vi "Init.vi"(8 "error in (no error)":errorcluster, 10 "RIO Device":T1="RIO0", 11 "AODAcq in":refnum<class "AODAcq.lvclass">) -> (0 "error out":errorcluster, 3 "AODAcq out":refnum<class "AODAcq.lvclass">)   [LabVIEW 2011, in "AODAcq.lvclass"]
uses:
  AODAcq.lvclass
  <vilib>/userdefined/High Color/nirio_resource_hc.ctl
  <vilib>/LabVIEW Targets/FPGA/RIO/nirio_PxiTriggers.ctl
  <vilib>/FPGAPlugInAG/PXIe-7965R/niLvFpga_Open_PXIe-7965R.vi
  <vilib>/FPGAPlugInAG/PXIe-7965R/niLvFpga_Reset_PXIe-7965R.vi
  <vilib>/FPGAPlugInAG/PXIe-7965R/niLvFpga_Run_PXIe-7965R.vi
  <vilib>/LabVIEW Targets/FPGA/RIO/nirioReserveTrigger.vi
  <vilib>/LabVIEW Targets/FPGA/79XXR/Private/79XXR_Method_IOModuleStatusImpl.vi
  <vilib>/Utility/error.llb/Error Cluster From Error Code.vi
  <vilib>/rvi/errors/niLvFpgaAdjustHostInterfaceError.vi
  <vilib>/rvi/interface/nirviOpenFPGA/nirviOpenFPGA.xnode
  FPGA_Control/AODRef.ctl
  FPGA_Control/FPGA Bitfiles/AODControl_FPGATarget_5751Acquire_F1CF9257.lvbitx
  FPGA_Control/AOD Control (FPGA).vi
  <vilib>/rvi/interface/nirviMethod/nirviMethod.xnode
  <vilib>/FPGA/interface/niFpgaViExecutionMode.ctl
  <vilib>/rvi/interface/nirviReadWriteControl/nirviReadWriteControl.xnode
  NiFpgaLv.dll
  <vilib>/FPGAPlugInAG/PXIe-7965R/niLvFpga_ConfigureFifo_PXIe-7965R.vi
  <vilib>/rvi/errors/niLvFpgaMergeErrorWithErrorCode.vi
  <vilib>/FPGAPlugInAG/PXIe-7965R/niLvFpga_StartFifo_PXIe-7965R.vi
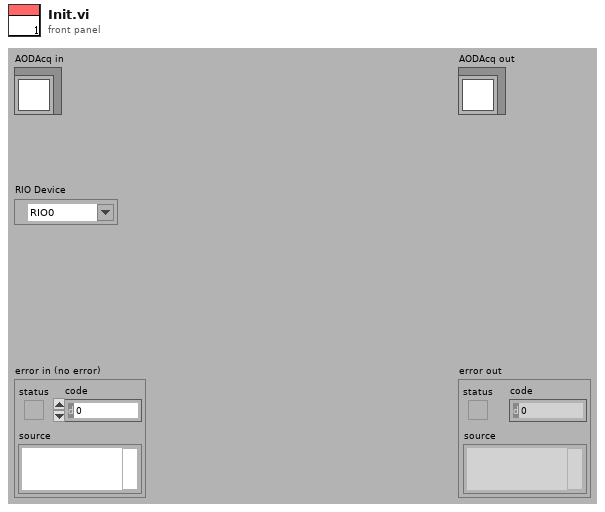
[diagram p1: front panel]
types:
  T1 = typedef "nirio_resource_hc.ctl" = tag
  T2 = typedef "AODRef.ctl" = refnum<k20>
  T3 = typedef "niFpgaViExecutionMode.ctl" = enum16{"FPGA Target", "Development Computer with Simulated I/O", "Development Computer with Real I/O", "Third-Party Simulator"}
  T4 = typedef "nirio_PxiTriggers.ctl" = u16
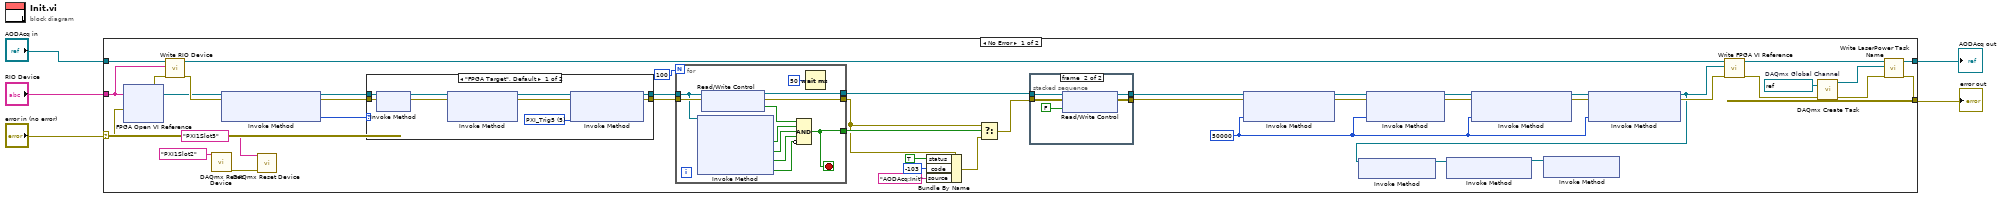
[diagram p0: block diagram]
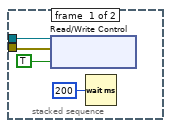
[diagram p2: hidden frame]
diagram:
  n1 = case shown="No Error" "error in (no error)" {
    selector: "error in (no error)" -> [w47 w82]
    tunnel: [w38 w82] -> w4
    tunnel: [w39 w81] -> w2
    tunnel: "AODAcq in" -> [w37 w81]
    tunnel: "RIO Device" -> [w35 _]
    frame No Error {
      w44 = refnum<k21> "AOD Gain"  # DAQmx Global Channel
      w12 = u32 50000 ("Depth")
      n2 = xnode "FPGA Open VI Reference"("error in"=w47, "resource name"=w35) -> ("FPGA VI Reference Out"=w32:T2, "error out"=w34:errorcluster)
      n3 = call-dynamic "Write RIO Device.vi"("error in (no error)"=w34, "RIO Device"=w35, "AODAcq in"=w37) -> ("error out"=w33:errorcluster, "AODAcq out"=w36:refnum<class "AODAcq.lvclass">)  [unwired: 7 in]
      n4 = call <vilib>:"DAQmx Reset Device.vi"("device in"=tag "PXI1Slot2") -> ("error out"=w19:errorcluster)  [unwired: 14 in]
      n5 = xnode "Invoke Method"("FPGA VI Reference In"=w32, "error in"=w33) -> ("FPGA VI Reference Out"=w49:T2, "error out"=w46:errorcluster, "FPGA VI Execution Mode"=w48:T3)
      n6 = call <vilib>:"DAQmx Reset Device.vi"("device in"=tag "PXI1Slot5", "error in"=w19) -> ()  [unwired: 13 in, 1 out]
      n7 = case shown="\"FPGA Target\", Default" w48 {
        tunnel: [w74 w80] -> w31
        tunnel: w49 -> [w78 w80]
        tunnel: w46 -> [w73 w79]
        tunnel: [w70 w79] -> w30
        frame "FPGA Target", Default {
          w76 = T4 5 items=["PXI_Trig0", "PXI_Trig1", "PXI_Trig2", "PXI_Trig3", "PXI_Trig4", "PXI_Trig5", "PXI_Trig6", "PXI_Trig7"] ("Trigger")
          n8 = xnode "Invoke Method"("FPGA VI Reference In"=w78, "error in"=w73) -> ("FPGA VI Reference Out"=w77:T2, "error out"=w72:errorcluster)
          n9 = xnode "Invoke Method"("FPGA VI Reference In"=w77, "error in"=w72) -> ("FPGA VI Reference Out"=w75:T2, "error out"=w71:errorcluster)  [unwired: 1 in]
          n10 = xnode "Invoke Method"("FPGA VI Reference In"=w75, "error in"=w71, "Trigger"=w76) -> ("FPGA VI Reference Out"=w74:T2, "error out"=w70:errorcluster)
        }
        frame "Development Computer with Simulated I/O" {
        }
      }
      n11 = for {
        N: 100 -> [_]
        tunnel: w31 -> [w59]
        tunnel: w30 -> [w60]
        tunnel: [w51] -> w29
        tunnel: [w53] -> w27
        tunnel: [w50] -> w22
        stop <- w51 stop-if-true
        n12 = xnode "Invoke Method"("FPGA VI Reference In"=w59) -> ("IO Module Present?"=w57:bool, "Power Enabled?"=w56:bool, "IO Enabled?"=w55:bool, "IO Module Mismatch?"=w54:bool)  [unwired: 1 in, 2 out]
        n13 = xnode "Read/Write Control"("FPGA VI Reference In"=w59, "error in"=w60) -> ("FPGA VI Reference Out"=w50:T2, "error out"=w53:errorcluster, "Status.Initialized"=w58:bool)
        n14 = Compound Arithmetic op=AND(w58, w57, w56, w55, invert w54) -> (w51:bool)
        n15 = Wait (ms)(milliseconds to wait=u32 50) -> ()  [unwired: 1 out]
      }
      n16 = Bundle By Name(cluster=w27, "status"=TRUE, "code"=-103, "source"="AODAcq:Init") -> (w26:errorcluster)
      n17 = Select(t=w27, s=w29, f=w26) -> (s? t:f=w21:errorcluster)
      n18 = stacked-sequence {
        tunnel: w22 -> [w64 w69]
        tunnel: w21 -> [w63 w68]
        tunnel: [_ w66] -> w7
        tunnel: [_ w65] -> w6
        frame #0 {
          n19 = xnode "Read/Write Control"("FPGA VI Reference In"=w64, "error in"=w63, "Control.Reset"=TRUE) -> ()  [unwired: 2 out]
          n20 = Wait (ms)(milliseconds to wait=u32 200) -> ()  [unwired: 1 out]
        }
        frame #1 {
          n21 = xnode "Read/Write Control"("FPGA VI Reference In"=w69, "error in"=w68, "Control.Reset"=FALSE) -> ("FPGA VI Reference Out"=w66:T2, "error out"=w65:errorcluster)
        }
      }
      n22 = xnode "Invoke Method"("FPGA VI Reference In"=w7, "error in"=w6, "Depth"=w12) -> ("FPGA VI Reference Out"=w11:T2, "error out"=w45:errorcluster)
      n23 = xnode "Invoke Method"("FPGA VI Reference In"=w11, "error in"=w45, "Depth"=w12) -> ("FPGA VI Reference Out"=w17:T2, "error out"=w16:errorcluster)
      n24 = xnode "Invoke Method"("FPGA VI Reference In"=w17, "error in"=w16, "Depth"=w12) -> ("FPGA VI Reference Out"=w15:T2, "error out"=w14:errorcluster)
      n25 = xnode "Invoke Method"("FPGA VI Reference In"=w15, "error in"=w14, "Depth"=w12) -> ("FPGA VI Reference Out"=w10:T2, "error out"=w13:errorcluster)
      n26 = xnode "Invoke Method"("FPGA VI Reference In"=w10) -> ("FPGA VI Reference Out"=w9:T2)  [unwired: 1 in, 1 out]
      n27 = xnode "Invoke Method"("FPGA VI Reference In"=w9) -> ("FPGA VI Reference Out"=w8:T2)  [unwired: 1 in, 1 out]
      n28 = xnode "Invoke Method"("FPGA VI Reference In"=w8) -> ()  [unwired: 1 in, 2 out]
      n29 = call-dynamic "Write FPGA VI Reference.vi"("error in (no error)"=w13, "AOD FPGA"=w10, "AODAcq in"=w36) -> ("error out"=w43:errorcluster, "AODAcq out"=w40:refnum<class "AODAcq.lvclass">)  [unwired: 7 in]
      n30 = call <vilib>:"DAQmx Create Task.vi"("global virtual channels"=w44, "error in"=w43) -> ("task out"=w41:refnum<k21>, "error out"=w42:errorcluster)  [unwired: 3 in, 9 out]
      n31 = call-dynamic "Write LaserPower Task Name.vi"("error in (no error)"=w42, "LaserPower Task Name"=w41, "AODAcq in"=w40) -> ("error out"=w38:errorcluster, "AODAcq out"=w39:refnum<class "AODAcq.lvclass">)  [unwired: 7 in]
    }
    frame Error {
    }
  }
  "error out" <- w4
  "AODAcq out" <- w2
